vi "GetColor.vi"(0 "CH":i32=1 min=1) -> (8 "Strings":string)   [LabVIEW 2017]
panel:
  in  "配列":string[](array[string])=["28,5,6", "0,13,23", "9,22,8", "21,0,21", "28,16,2", "5,23,30", "30,23,1", "28,0,17", "17,11,7", "19,27,0"]
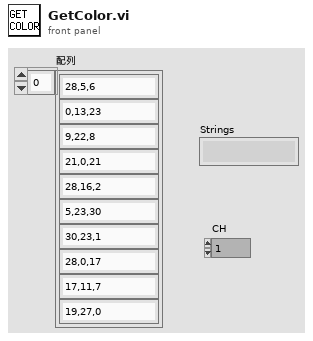
[diagram p1: front panel]
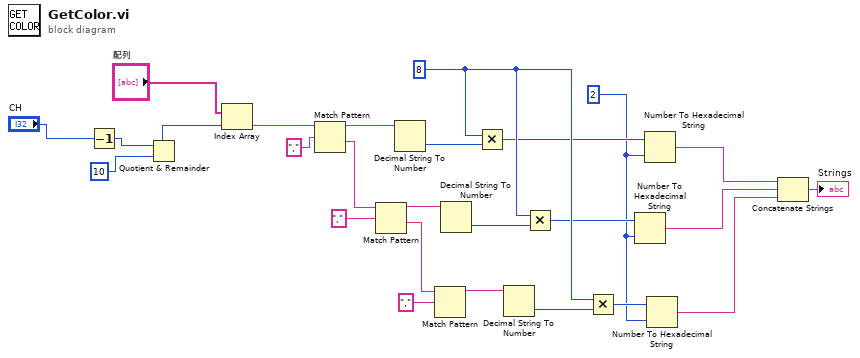
[diagram p0: block diagram]
diagram:
  w5 = 2
  w13 = 8
  n1 = Decrement(x="CH") -> (x-1=w2:i32)
  n2 = Quotient & Remainder(x=w2, y=10) -> (x-y*floor(x/y)=w26:i32)  [unwired: 1 out]
  n3 = Index Array(array="配列", index=w26) -> (element=w4:string)
  n4 = Match Pattern(string=w4, regular expression="," ("正規表現")) -> (before substring=w23:string, after substring=w19:string)  [unwired: 1 in, 2 out]
  n5 = Match Pattern(string=w19, regular expression="," ("正規表現")) -> (before substring=w16:string, after substring=w18:string)  [unwired: 1 in, 2 out]
  n6 = Decimal String To Number(string=w23) -> (number=w22:i32)  [unwired: 2 in, 1 out]
  n7 = Match Pattern(string=w18, regular expression="," ("正規表現")) -> (before substring=w14:string)  [unwired: 1 in, 3 out]
  n8 = Decimal String To Number(string=w16) -> (number=w17:i32)  [unwired: 2 in, 1 out]
  n9 = Multiply(x=w13, y=w22) -> (x*y=w12:i32)
  n10 = Decimal String To Number(string=w14) -> (number=w15:i32)  [unwired: 2 in, 1 out]
  n11 = Multiply(x=w13, y=w17) -> (x*y=w11:i32)
  n12 = Multiply(x=w13, y=w15) -> (x*y=w10:i32)
  n13 = Number To Hexadecimal String(1:w5, 2:w11) -> (0:w8:string)
  n14 = Number To Hexadecimal String(1:w5, 2:w12) -> (0:w9:string)
  n15 = Number To Hexadecimal String(1:w5, 2:w10) -> (0:w7:string)
  n16 = Concatenate Strings(w9, w8, w7) -> (→"Strings":string)
